vi "Initialize From Config.vi"(0 "Engine Data":T1={"Loop Info"={"Processor"=-2, "Priority"=0}, "Main Tag Data"={"Double"=[], "Single"=[], "I64"=[], "I32"=[], "I16"=[], "I8"=[], "U64"=[], "U32"=[], "U16"=[], "U8"=[], "Boolean"=[], "String"=[], "Array of Double"=[], "Array of Single"=[], "Array of I64"=[], "Array of I32"=[], "Array of I16"=[], "Array of I8"=[], "Array of U64"=[], "Array of U32"=[], "Array of U16"=[], "Array of U8"=[], "Array of Boolean"=[], "Array of String"=[]}, "Module Info"={"Tag Bus Modules"=[], "Execute?"=[], "Input Method Indices"=[], "Process Method Indices"=[], "Output Method Indices"=[], "Input Transfer Specifications"=[], "Parameter Transfer Specifications"=[], "Result Transfer Specifications"=[], "Output Transfer Specifications"=[], "Module Errors"=[], "Module Decimation"=[], "Module Decimation Indices"=[], "Error Queue"=refnum, "Module Error Configuration"=[], "Module Errors (n-1)"=[]}, "engine timing source"=refnum, "timing policy"=enum."nonblocking", "async execution info"={"Tag Bus Modules"=[], "Execute?"=[], "Input Method Indices"=[], "Process Method Indices"=[], "Output Method Indices"=[], "Input Transfer Specifications"=[], "Parameter Transfer Specifications"=[], "Result Transfer Specifications"=[], "Output Transfer Specifications"=[], "Module Errors"=[], "Module Decimation"=[], "Module Decimation Indices"=[], "Error Queue"=refnum, "Module Error Configuration"=[], "comm errors"=[], "Module Errors (n-1)"=[]}, "status reporting"={"late index (bool)"=-1, "late count (U32)"=-1, "current dt ns(U64)"=-1, "synchronous modules"=[], "asynchronous modules"=[]}}, 5 "Engine Configuration":refnum<class "Standard Engine Configuration.lvclass">, 7 "Modules":refnum<class "TBM module execution interface.lvclass">[](array[class]), 9 "Module Configurations":refnum<class "TBM module configuration.lvclass">[](array[class]), 11 "error in":errorcluster) -> (4 "Engine Data Out":T1={"Loop Info"={"Processor"=-2, "Priority"=0}, "Main Tag Data"={"Double"=[], "Single"=[], "I64"=[], "I32"=[], "I16"=[], "I8"=[], "U64"=[], "U32"=[], "U16"=[], "U8"=[], "Boolean"=[], "String"=[], "Array of Double"=[], "Array of Single"=[], "Array of I64"=[], "Array of I32"=[], "Array of I16"=[], "Array of I8"=[], "Array of U64"=[], "Array of U32"=[], "Array of U16"=[], "Array of U8"=[], "Array of Boolean"=[], "Array of String"=[]}, "Module Info"={"Tag Bus Modules"=[], "Execute?"=[], "Input Method Indices"=[], "Process Method Indices"=[], "Output Method Indices"=[], "Input Transfer Specifications"=[], "Parameter Transfer Specifications"=[], "Result Transfer Specifications"=[], "Output Transfer Specifications"=[], "Module Errors"=[], "Module Decimation"=[], "Module Decimation Indices"=[], "Error Queue"=refnum, "Module Error Configuration"=[], "Module Errors (n-1)"=[]}, "engine timing source"=refnum, "timing policy"=enum."nonblocking", "async execution info"={"Tag Bus Modules"=[], "Execute?"=[], "Input Method Indices"=[], "Process Method Indices"=[], "Output Method Indices"=[], "Input Transfer Specifications"=[], "Parameter Transfer Specifications"=[], "Result Transfer Specifications"=[], "Output Transfer Specifications"=[], "Module Errors"=[], "Module Decimation"=[], "Module Decimation Indices"=[], "Error Queue"=refnum, "Module Error Configuration"=[], "comm errors"=[], "Module Errors (n-1)"=[]}, "status reporting"={"late index (bool)"=-1, "late count (U32)"=-1, "current dt ns(U64)"=-1, "synchronous modules"=[], "asynchronous modules"=[]}}, 15 "error out":errorcluster)   [LabVIEW 2013, in "Standard Engine Runtime.lvclass"]
uses:
  Standard Engine Runtime.lvclass
  Engine Data.ctl
  <vilib>/NI/Module Timing Source/timing source/TBM timing source.lvclass
  Configuration/Loop Info.ctl
  <vilib>/NI/Tag Bus/table/data table.ctl
  Module Execution Info.ctl
  <vilib>/NI/Tag Bus Module Framework/runtime/TBM module execution interface.lvclass
  Data Table with Transfer Spec.ctl
  <vilib>/NI/Tag Bus/table/transfer specification.ctl
  <vilib>/NI/Tag Bus/tag/Data Type.ctl
  Configuration/Module Decimation.ctl
  Configuration/Module Error Configuration.ctl
  Configuration/Error Actions By Category.ctl
  <vilib>/NI/Tag Bus Module Framework/runtime/error classification.ctl
  Configuration/Error Actions.ctl
  Configuration/timing policy.ctl
  async execution info.ctl
  asynchronous process data.ctl
  async command notification.ctl
  <vilib>/NI/Tag Bus Module Framework/runtime/execution settings.ctl
  async error info.ctl
  status reporting data.ctl
  module status reporting.ctl
  Configuration/Standard Engine Configuration.lvclass
  <vilib>/NI/Tag Bus Module Framework/module configuration/TBM module configuration.lvclass
  Configuration/Standard Engine Configuration.lvclass/Standard Engine Configuration.ctl
  <vilib>/NI/Tag Bus Module Framework/root configuration/TBM configuration.lvclass/TBM configuration.ctl
  <vilib>/NI/Module Timing Source/standard timing source/ms timing source.lvclass
  <vilib>/NI/Module Timing Source/usec timing source/usec timing source.lvclass
  <vilib>/NI/Module Timing Source/scan engine timing source/scan engine timing source.lvclass
  <vilib>/NI/Module Timing Source/timing source/TBM timing source.lvclass/TBM timing source.ctl
  <vilib>/NI/Module Execution Interface/Engine Configuration/engine configuration.lvclass/engine configuration.ctl
  <vilib>/NI/Tag Bus/dictionary/data dictionary.lvclass/data dictionary.ctl
  <vilib>/NI/Tag Bus/dictionary/lookup polymorphs/locate I32.vi
  Configuration/Read timing policy.vi
  Configuration/Read Timing Source Type.vi
  Configuration/Read Processor.vi
  Configuration/Read Master Timing Module.vi
  <vilib>/NI/Tag Bus/dictionary/search/find data index.vi
  <vilib>/NI/Tag Bus/dictionary/search/search string list.vi
  Configuration/Read Timing Source dt.vi
  <vilib>/NI/Tag Bus Module Framework/root configuration/create GUID.vi
  Configuration/Find Module Specific Config.vi
  <vilib>/Utility/error.llb/Error Cluster From Error Code.vi
  <vilib>/NI/Tag Bus/dictionary/tag not found.vi
  <vilib>/NI/Tag Bus/tag/tag descriptor.lvclass
  <vilib>/Utility/RT CPU pool selections.ctl
  <vilib>/NI/Tag Bus/dictionary/data dictionary.lvclass
  <vilib>/NI/Module Execution Interface/Engine Configuration/engine configuration.lvclass
  <vilib>/NI/Module Execution Interface/Engine Runtime/Engine Runtime Interface.lvclass
  <vilib>/NI/Tag Bus Module Framework/root configuration/TBM configuration.lvclass
  <vilib>/NI/Tag Bus/table/data table.lvlib
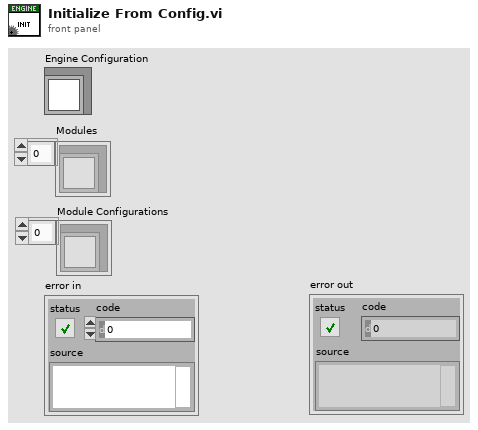
[diagram p1: front panel]
types:
  T1 = typedef "Standard Engine Runtime.lvclass/Engine Data.ctl" = cluster{"Loop Info":T2, "Main Tag Data":T3, "Module Info":T4, "engine timing source":refnum<class "TBM timing source.lvclass">, "timing policy":T13, "async execution info":T14, "status reporting":T17}
  T2 = typedef "Standard Engine Configuration.lvclass/Loop Info.ctl" = cluster{"Processor":i32, "Priority":i32}
  T3 = typedef "tag bus.lvlib/data table.lvlib/data table.ctl" = cluster{"Double":dbl[], "Single":sgl[], "I64":i64[], "I32":i32[], "I16":i16[], "I8":i8[], "U64":u64[], "U32":u32[], "U16":u16[], "U8":u8[], "Boolean":bool[], "String":string[], "Array of Double":cluster{"DBL Array":dbl[]}[], "Array of Single":cluster{"SGL Array":sgl[]}[], "Array of I64":cluster{"I64 Array":i64[]}[], "Array of I32":cluster{"I32 Array":i32[]}[], "Array of I16":cluster{"I16 Array":i16[]}[], "Array of I8":cluster{"I8 Array":i8[]}[], "Array of U64":cluster{"U64 Array":u64[]}[], "Array of U32":cluster{"U32 Array":u32[]}[], "Array of U16":cluster{"U16 Array":u16[]}[], "Array of U8":cluster{"U8 Array":u8[]}[], "Array of Boolean":cluster{"Boolean Array":bool[]}[], "Array of String":cluster{"String Array":string[]}[]}
  T4 = typedef "Standard Engine Runtime.lvclass/Module Execution Info.ctl" = cluster{"Tag Bus Modules":refnum<class "TBM module execution interface.lvclass">[], "Execute?":bool[], "Input Method Indices":i32[], "Process Method Indices":i32[], "Output Method Indices":i32[], "Input Transfer Specifications":T5[], "Parameter Transfer Specifications":T5[], "Result Transfer Specifications":T5[], "Output Transfer Specifications":T5[], "Module Errors":errorcluster[], "Module Decimation":T8[], "Module Decimation Indices":i32[], "Error Queue":refnum<queue>, "Module Error Configuration":T9[], "Module Errors (n-1)":errorcluster[]}
  T5 = typedef "Standard Engine Runtime.lvclass/Data Table with Transfer Spec.ctl" = cluster{"Data Table":T3, "Transfer Specification":T6[]}
  T6 = typedef "tag bus.lvlib/data table.lvlib/transfer specification.ctl" = cluster{"data type":T7, "sink indices":i32[], "source indices":i32[]}
  T7 = typedef "tag bus.lvlib/tag descriptor.lvclass/Data Type.ctl" = enum16{"Double", "Single", "I64", "I32", "I16", "I8", "U64", "U32", "U16", "U8", "Boolean", "String", "Array of Double", "Array of Single", "Array of I64", "Array of I32", "Array of I16", "Array of I8", "Array of U64", "Array of U32", "Array of U16", "Array of U8", "Array of Boolean", "Array of String"}
  T8 = typedef "Standard Engine Configuration.lvclass/Module Decimation.ctl" = cluster{"Decimation":u16, "Offset":u16}
  T9 = typedef "Standard Engine Configuration.lvclass/Module Error Configuration.ctl" = cluster{"Module Error Configuration":T10[]}
  T10 = typedef "Standard Engine Configuration.lvclass/Error Actions By Category.ctl" = cluster{"error classification":T11, "Error Actions":T12[]}
  T11 = typedef "TBM module execution interface.lvclass/error classification.ctl" = enum16{"unknown", "none", "trivial", "recoverable", "critical"}
  T12 = typedef "Standard Engine Configuration.lvclass/Error Actions.ctl" = enum16{"Clear", "Notify", "Stop Component", "Stop Engine", "Safe State", "Attempt Recovery"}
  T13 = typedef "Standard Engine Configuration.lvclass/timing policy.ctl" = enum16{"strict determinism", "nonblocking", "nondeterministic inline"}
  T14 = typedef "Standard Engine Runtime.lvclass/async execution info.ctl" = cluster{"Tag Bus Modules":T15[], "Execute?":bool[], "Input Method Indices":i32[], "Process Method Indices":i32[], "Output Method Indices":i32[], "Input Transfer Specifications":T5[], "Parameter Transfer Specifications":T5[], "Result Transfer Specifications":T5[], "Output Transfer Specifications":T5[], "Module Errors":errorcluster[], "Module Decimation":T8[], "Module Decimation Indices":i32[], "Error Queue":refnum<queue>, "Module Error Configuration":T9[], "comm errors":errorcluster[], "Module Errors (n-1)":errorcluster[]}
  T15 = typedef "Standard Engine Runtime.lvclass/asynchronous process data.ctl" = cluster{"thread reference":refnum<vi>, "cmd notification":refnum<k33>, "execution period (ms)":i32, "input from component":refnum<queue>, "input to component":refnum<queue>, "output from component":refnum<queue>, "output to component":refnum<queue>, "process input from component":refnum<queue>, "process input to component":refnum<queue>, "process result from component":refnum<queue>, "process result to component":refnum<queue>, "execution settings":T16, "error fifo":refnum<k33>}
  T16 = typedef "TBM module execution interface.lvclass/execution settings.ctl" = cluster{"reads inputs":bool, "processes data":bool, "writes outputs":bool}
  T17 = typedef "Standard Engine Runtime.lvclass/status reporting data.ctl" = cluster{"late index (bool)":i32, "late count (U32)":i32, "current dt ns(U64)":i32, "synchronous modules":T18[], "asynchronous modules":T18[]}
  T18 = typedef "Standard Engine Runtime.lvclass/module status reporting.ctl" = cluster{"module index":i32, "error tag (I32)":i32}
  T19 = typedef "Standard Engine Configuration.lvclass/Supported Timing Sources.ctl" = enum16{"Use Module Timing Source", "1 kHz Clock", "1 MHz Clock", "Synchronize to Scan Engine"}
  T20 = cluster{"execution order priority":i32, "module index":i32}
  T21 = typedef "engine configuration.lvclass/Module Mappings.ctl" = cluster{"Owning ID":string, "Input Mappings":T22[], "Process Parameter Mappings":T22[], "Process Results Mappings":T22[], "Output Mappings":T22[]}
  T22 = typedef "tag bus.lvlib/data table.lvlib/mapping specification.ctl" = cluster{"data type":T7, "mappings":T23[]}
  T23 = typedef "tag bus.lvlib/data table.lvlib/mapping.ctl" = cluster{"sink name":string, "source name":string}
  T24 = typedef "TBM channel.lvclass/data tables.ctl" = cluster{"input data":T25, "processing parameter":T25, "processing result":T25, "output data":T25}
  T25 = typedef "tag bus.lvlib/dictionary table pair.ctl" = cluster{"data dictionary":refnum<class "data dictionary.lvclass">, "data table":T3}
  T26 = typedef "Standard Engine Configuration.lvclass/timing reporting tags.ctl" = cluster{"late index (bool)":string, "late count index (U32)":string, "current dt ns(U64)":string}
  T27 = typedef "NI_Real-Time Target Support.lvlib/RT CPU pool selections.ctl" = enum16{"System & Timed Structures", "System", "Timed Structures", "Reserved"}
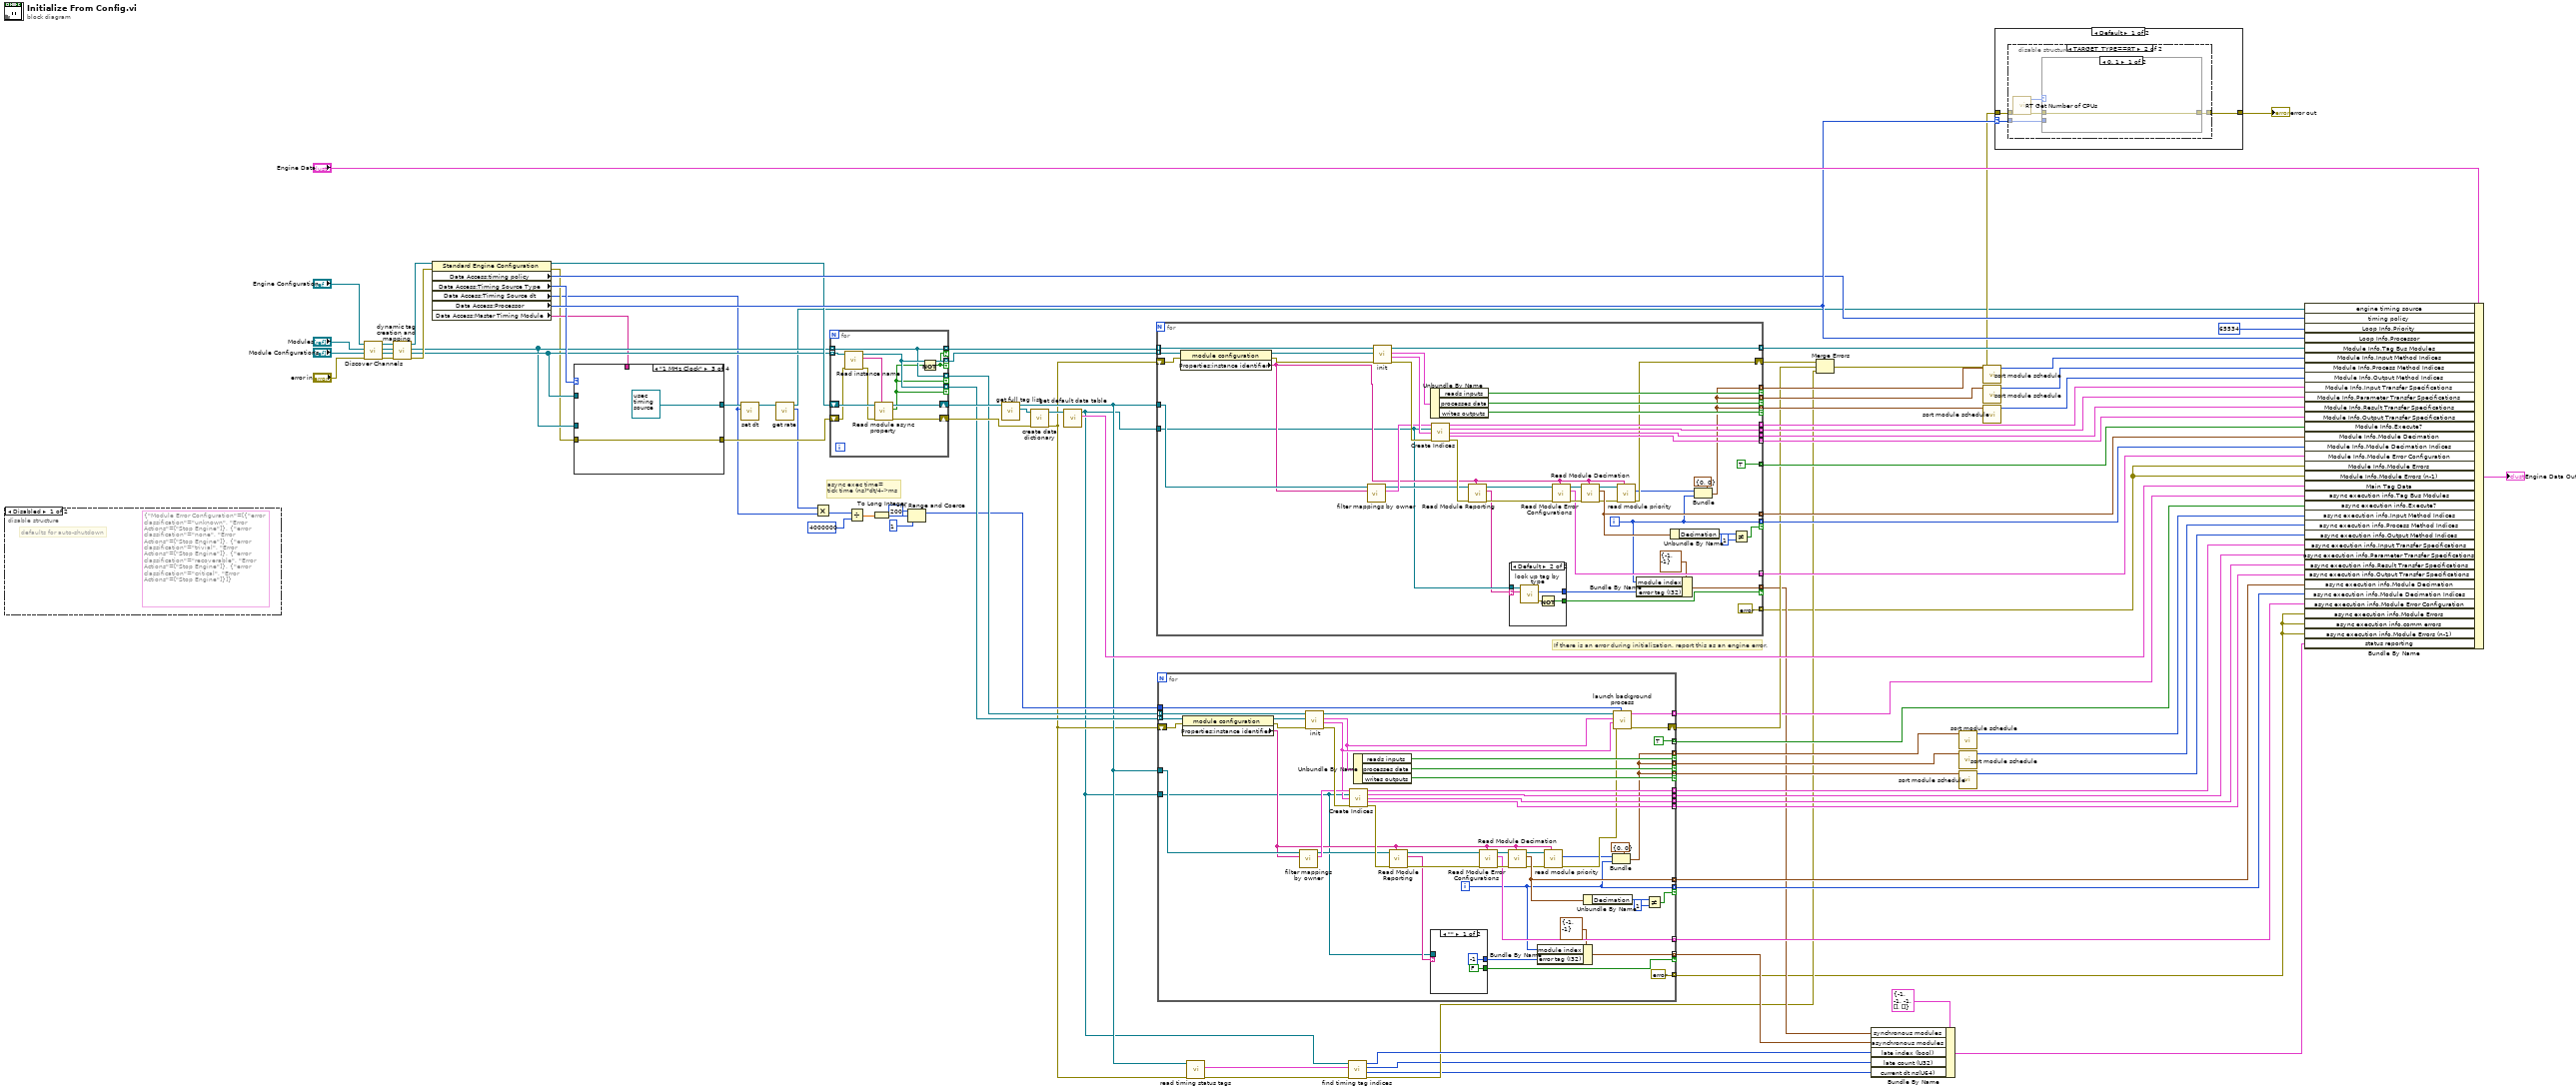
[diagram p0: block diagram]
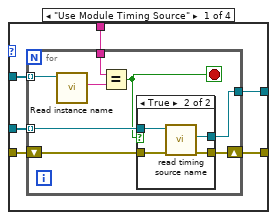
[diagram p2: hidden frame]
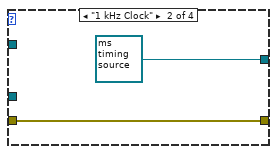
[diagram p4: hidden frame]
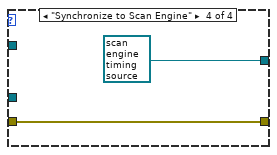
[diagram p5: hidden frame]
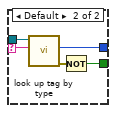
[diagram p6: hidden frame]
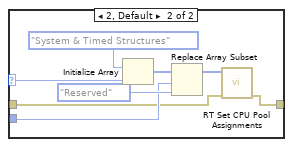
[diagram p9: hidden frame]
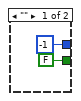
[diagram p11: hidden frame]
diagram:
  # "async exec time=\ntick time (ns)*dt/4->ms"
  # "If there is an error during initialization, report this as an engine error."
  n1 = disable-structure shown="Disabled" {
    frame Disabled {
      (unwired) T9 {"Module Error Configuration"=[{"error classification"=enum."unknown", "Error Actions"=[enum."Stop Engine"]}, {"error classification"=enum."none", "Error Actions"=[enum."Stop Engine"]}, {"error classification"=enum."trivial", "Error Actions"=[enum."Stop Engine"]}, {"error classification"=enum."recoverable", "Error Actions"=[enum."Stop Engine"]}, {"error classification"=enum."critical", "Error Actions"=[enum."Stop Engine"]}]} ("Module Error Configuration")
      # "defaults for auto-shutdown"
    }
    frame Enabled {
    }
  }
  n2 = call <vilib>:"Discover Channels.vi"("error in (no error)"="error in", "module configurations"="Module Configurations", "modules"="Modules", "engine configuration"="Engine Configuration") -> ("error out"=w76:errorcluster, "module configurations out"=w77:refnum<class "TBM module configuration.lvclass">[], "modules out"=w78:refnum<class "TBM module execution interface.lvclass">[], "engine configuration out"=w79:refnum<class "Standard Engine Configuration.lvclass">)  [unwired: 4 in]
  n3 = call <vilib>:"dynamic tag creation and mapping.vi"("error in"=w76, "module configurations"=w77, "modules"=w78, "engine configuration in"=w79) -> ("error out"=w70:errorcluster, "module configurations out"=w32:refnum<class "TBM module configuration.lvclass">[], "modules out"=w31:refnum<class "TBM module execution interface.lvclass">[], "engine configuration out"=w71:refnum<class "Standard Engine Configuration.lvclass">)  [unwired: 4 in]
  n4 = property class="Standard Engine Configuration"(reference=w71, error in=w70) -> (reference out=w57:refnum<class "Standard Engine Configuration.lvclass">, error out=w28:errorcluster, "Data Access:timing policy"=w58:T13, "Data Access:Timing Source Type"=w33:T19, "Data Access:Timing Source dt"=w23:u32, "Data Access:Processor"=w65:i32, "Data Access:Master Timing Module"=w30:string)
  n5 = case shown="\"1 MHz Clock\"" w33 {
    tunnel: [w95 refnum<class "ms timing source.lvclass"> refnum ("ms timing source.lvclass") refnum<class "usec timing source.lvclass"> refnum ("usec timing source.lvclass") refnum<class "scan engine timing source.lvclass"> refnum ("scan engine timing source.lvclass")] -> w27
    tunnel: w32 -> [w98 _ _ _]
    tunnel: w31 -> [w97 _ _ _]
    tunnel: w30 -> [w96 _ _ _]
    tunnel: [w94 w112 w114 w116] -> w29
    tunnel: w28 -> [w93 w112 w114 w116]
    frame "Use Module Timing Source" {
      n6 = for {
        tunnel: w98 -> [w106] mode=indexing
        tunnel: w97 -> [w103] mode=indexing
        tunnel: w96 -> [w104]
        tunnel: [w101] -> w95
        shift-right: [w100] -> w94
        shift-left: w93 -> [w99]
        stop <- w102 stop-if-true
        n7 = call <vilib>:"Read instance name.vi"("configuration in"=w106) -> ("instance id"=w105:string)  [unwired: 8 in, 2 out]
        n8 = Equal?(x=w104, y=w105) -> (x = y?=w102:bool)
        n9 = case shown="True" w102 {
          tunnel: w103 -> [_ w111]
          tunnel: [_ w110] -> w101
          tunnel: [w107 w109] -> w100
          tunnel: w99 -> [w107 w108]
          frame False {
          }
          frame True {
            n10 = call-dynamic "read timing source name.vi"("error in"=w108, "module in"=w111) -> ("error out"=w109:errorcluster, "timing source"=w110:refnum<class "TBM timing source.lvclass">)  [unwired: 7 in, 1 out]
          }
        }
      }
    }
    frame "1 kHz Clock" {
    }
    frame "1 MHz Clock" {
    }
    frame "Synchronize to Scan Engine" {
    }
  }
  n11 = call <vilib>:"set dt.vi"("dt"=w23, "timing source in"=w27) -> ("timing source out"=w26:refnum<class "TBM timing source.lvclass">)  [unwired: 9 in]
  n12 = call-dynamic "get rate.vi"("timing source in"=w26) -> ("period (ns)"=w24:i64, "timing source out"=w25:refnum<class "TBM timing source.lvclass">)  [unwired: 8 in, 1 out]
  n13 = Multiply(x=w24, y=w23) -> (x*y=w22:i64)
  n14 = for {
    tunnel: w32 -> [w128] mode=indexing
    tunnel: w31 -> [w123] mode=indexing
    shift-right: [w125] -> w56
    shift-left: w57 -> [w126]
    tunnel: [w124] -> w54 mode=indexing if=w119
    tunnel: [w123] -> w55 mode=indexing if=w119
    tunnel: [w124] -> w51 mode=indexing if=w118
    tunnel: [w123] -> w52 mode=indexing if=w118
    shift-right: [w122] -> w53
    shift-left: w29 -> [w120]
    n15 = call <vilib>:"Read instance name.vi"("error in"=w120, "configuration in"=w128) -> ("error out"=w121:errorcluster, "instance id"=w127:string, "configuration out"=w124:refnum<class "TBM module configuration.lvclass">)  [unwired: 7 in]
    n16 = call "Read module async property.vi"("Module ID"=w127, "error in"=w121, "Standard Engine Repo Data in"=w126) -> ("error out"=w122:errorcluster, "async?"=w118:bool, "Standard Engine Repo Data out"=w125:refnum<class "Standard Engine Configuration.lvclass">)  [unwired: 6 in]
    n17 = Not(x=w118) -> (.not. x?=w119:bool)
  }
  n18 = Divide(x=w22, y=i64 4000000) -> (x/y=w20:dbl)
  n19 = To Long Integer(number=w20) -> (32bit integer=w19:i32)
  n20 = In Range and Coerce(upper limit=200, x=w19, lower limit=1) -> (coerced(x)=w18:i32)  [unwired: 1 out]
  n21 = call <vilib>:"get full tag list.vi"("engine configuration in"=w56) -> ("tag list"=w69:refnum<class "tag descriptor.lvclass">[], "engine configuration out"=w11:refnum<class "Standard Engine Configuration.lvclass">)  [unwired: 9 in]
  n22 = call <vilib>:"create data dictionary.vi"("error in"=w53, "system tags"=w69) -> ("error out"=w10:errorcluster, "data dictionary"=w68:refnum<class "data dictionary.lvclass">)  [unwired: 8 in]
  n23 = call <vilib>:"get default data table.vi"("data dictionary in"=w68) -> ("default data table"=w80:T3, "data dictionary out"=w7:refnum<class "data dictionary.lvclass">)  [unwired: 9 in]
  n24 = for {
    tunnel: w54 -> [w158] mode=indexing
    shift-right: [w147] -> w84
    shift-left: w10 -> [w154]
    tunnel: w55 -> [w173] mode=indexing
    tunnel: [w152] -> w92 mode=indexing
    tunnel: [w144] -> w59 mode=indexing if=w172
    tunnel: [w144] -> w62 mode=indexing if=w171
    tunnel: [w144] -> w64 mode=indexing if=w170
    tunnel: [w169] -> w90 mode=indexing
    tunnel: [w168] -> w89 mode=indexing
    tunnel: [w167] -> w88 mode=indexing
    tunnel: [w166] -> w87 mode=indexing
    tunnel: [TRUE] -> w86 mode=indexing
    tunnel: [w133] -> w85 mode=indexing if=w162
    tunnel: [w149] -> w81 mode=indexing
    tunnel: [w157] -> w82 mode=indexing
    tunnel: [errorcluster {"status"=FALSE, "code"=0, "source"=""} ("error constant")] -> w2 mode=indexing
    tunnel: w7 -> [w132]
    tunnel: w11 -> [w141]
    tunnel: [w134] -> w14 mode=indexing if=w130
    i -> [w133]
    n25 = property class="module configuration"(reference=w158, error in=w154) -> (reference out=w155:refnum<class "TBM module configuration.lvclass">, error out=w142:errorcluster, "Properties:instance identifier"=w136:string)
    n26 = call <vilib>:"filter mappings by owner.vi"("owner"=w136, "engine configuration in"=w141) -> ("module mapping"=w153:T21, "engine configuration out"=w139:refnum<class "Standard Engine Configuration.lvclass">)  [unwired: 8 in]
    n27 = call-dynamic "init.vi"("error in"=w142, "module configuration"=w155, "module in"=w173) -> ("error out"=w165:errorcluster, "data allocations"=w159:T24, "execution settings"=w160:T16, "module out"=w152:refnum<class "TBM module execution interface.lvclass">)  [unwired: 5 in]
    n28 = Unbundle By Name(w160) -> ("reads inputs"=w172:bool, "processes data"=w171:bool, "writes outputs"=w170:bool)
    n29 = call "Create Indices.vi"("Component Mappings"=w153, "main data dictionary"=w132, "data description"=w159, "error in"=w165) -> ("Input Transfer Specification"=w169:T5, "Parameter Transfer Specifcation"=w168:T5, "Result Transfer Specifcation"=w167:T5, "Output Transfer Specifcation"=w166:T5, "error out"=w140:errorcluster)  [unwired: 7 in]
    n30 = call "Read Module Reporting.vi"("Module ID"=w136, "error in"=w140, "Standard Engine Repo Data in"=w139) -> ("error out"=w138:errorcluster, "error tag"=w129:string, "Standard Engine Repo Data out"=w137:refnum<class "Standard Engine Configuration.lvclass">)  [unwired: 6 in]
    n31 = case shown="Default" w129 {
      selector: w129 -> [_ w176]
      tunnel: w132 -> [_ w180]
      tunnel: [-1 ("index") w179] -> w131
      tunnel: [FALSE w177] -> w130
      frame "" {
      }
      frame Default {
        n32 = call-poly <vilib>:"look up tag by type.vi"("name"=w176, "data dictionary in"=w180) -> ("error out"=w178:errorcluster, "index"=w179:i32)  [unwired: 7 in, 1 out]
        n33 = Not(x=w178) -> (.not. x?=w177:bool)
      }
    }
    n34 = call "Read Module Error Configurations.vi"("Module ID"=w136, "error in"=w138, "Standard Engine Repo Data in"=w137) -> ("error out"=w150:errorcluster, "Module Error Configuration"=w149:T9, "Standard Engine Repo Data out"=w151:refnum<class "Standard Engine Configuration.lvclass">)  [unwired: 6 in]
    n35 = call "Read Module Decimation.vi"("Module ID"=w136, "error in"=w150, "Standard Engine Repo Data in"=w151) -> ("error out"=w148:errorcluster, "Module Decimation"=w157:T8, "Standard Engine Repo Data out"=w146:refnum<class "Standard Engine Configuration.lvclass">)  [unwired: 6 in]
    n36 = call "read module priority.vi"("Module ID"=w136, "error in"=w148, "Standard Engine Repo Data in"=w146) -> ("error out"=w147:errorcluster, "execution order priority"=w145:i32)  [unwired: 6 in, 1 out]
    n37 = Bundle By Name(cluster=T18 {"module index"=-1, "error tag (I32)"=-1} ("module status report"), "module index"=w133, "error tag (I32)"=w131) -> (w134:T18)
    n38 = Unbundle By Name(w157) -> ("Decimation"=w156:u16)
    n39 = Bundle(cluster=T20 {"execution order priority"=0, "module index"=0} ("priority cluster"), "execution order priority"=w145, "module index"=w133) -> (w144:T20)
    n40 = Not Equal?(x=w156, y=u16 1) -> (x != y?=w162:bool)
  }
  n41 = for {
    tunnel: w51 -> [w215] mode=indexing
    shift-right: [w197] -> w48
    shift-left: w10 -> [w211]
    tunnel: w52 -> [w228] mode=indexing
    tunnel: [w201] -> w45 mode=indexing if=w227
    tunnel: [w201] -> w46 mode=indexing if=w226
    tunnel: [w201] -> w47 mode=indexing if=w225
    tunnel: [w224] -> w40 mode=indexing
    tunnel: [w223] -> w39 mode=indexing
    tunnel: [w222] -> w38 mode=indexing
    tunnel: [w221] -> w37 mode=indexing
    tunnel: [TRUE] -> w43 mode=indexing
    tunnel: [w181] -> w35 mode=indexing if=w217
    tunnel: [w206] -> w50 mode=indexing
    tunnel: [w214] -> w36 mode=indexing
    tunnel: [errorcluster {"status"=FALSE, "code"=0, "source"=""} ("error constant")] -> w1 mode=indexing
    tunnel: w7 -> [w182]
    tunnel: w11 -> [w199]
    tunnel: [w196] -> w34 mode=indexing
    tunnel: w18 -> [w193]
    tunnel: [w186] -> w13 mode=indexing if=w184
    i -> [w181]
    n42 = property class="module configuration"(reference=w215, error in=w211) -> (reference out=w212:refnum<class "TBM module configuration.lvclass">, error out=w198:errorcluster, "Properties:instance identifier"=w188:string)
    n43 = call <vilib>:"filter mappings by owner.vi"("owner"=w188, "engine configuration in"=w199) -> ("module mapping"=w210:T21, "engine configuration out"=w190:refnum<class "Standard Engine Configuration.lvclass">)  [unwired: 8 in]
    n44 = call-dynamic "init.vi"("error in"=w198, "module configuration"=w212, "module in"=w228) -> ("error out"=w220:errorcluster, "data allocations"=w195:T24, "execution settings"=w194:T16, "module out"=w209:refnum<class "TBM module execution interface.lvclass">)  [unwired: 5 in]
    n45 = call "Create Indices.vi"("Component Mappings"=w210, "main data dictionary"=w182, "data description"=w195, "error in"=w220) -> ("Input Transfer Specification"=w224:T5, "Parameter Transfer Specifcation"=w223:T5, "Result Transfer Specifcation"=w222:T5, "Output Transfer Specifcation"=w221:T5, "error out"=w192:errorcluster)  [unwired: 7 in]
    n46 = Unbundle By Name(w194) -> ("reads inputs"=w227:bool, "processes data"=w226:bool, "writes outputs"=w225:bool)
    n47 = call "Read Module Reporting.vi"("Module ID"=w188, "error in"=w192, "Standard Engine Repo Data in"=w190) -> ("error out"=w191:errorcluster, "error tag"=w183:string, "Standard Engine Repo Data out"=w189:refnum<class "Standard Engine Configuration.lvclass">)  [unwired: 6 in]
    n48 = case shown="\"\"" w183 {
      selector: w183 -> [_ w231]
      tunnel: w182 -> [_ w235]
      tunnel: [-1 ("index") w234] -> w185
      tunnel: [FALSE w232] -> w184
      frame "" {
      }
      frame Default {
        n49 = call-poly <vilib>:"look up tag by type.vi"("name"=w231, "data dictionary in"=w235) -> ("error out"=w233:errorcluster, "index"=w234:i32)  [unwired: 7 in, 1 out]
        n50 = Not(x=w233) -> (.not. x?=w232:bool)
      }
    }
    n51 = call "Read Module Error Configurations.vi"("Module ID"=w188, "error in"=w191, "Standard Engine Repo Data in"=w189) -> ("error out"=w207:errorcluster, "Module Error Configuration"=w206:T9, "Standard Engine Repo Data out"=w208:refnum<class "Standard Engine Configuration.lvclass">)  [unwired: 6 in]
    n52 = call "Read Module Decimation.vi"("Module ID"=w188, "error in"=w207, "Standard Engine Repo Data in"=w208) -> ("error out"=w205:errorcluster, "Module Decimation"=w214:T8, "Standard Engine Repo Data out"=w203:refnum<class "Standard Engine Configuration.lvclass">)  [unwired: 6 in]
    n53 = Bundle By Name(cluster=T18 {"module index"=-1, "error tag (I32)"=-1} ("module status report"), "module index"=w181, "error tag (I32)"=w185) -> (w186:T18)
    n54 = call "read module priority.vi"("Module ID"=w188, "error in"=w205, "Standard Engine Repo Data in"=w203) -> ("error out"=w204:errorcluster, "execution order priority"=w202:i32)  [unwired: 6 in, 1 out]
    n55 = Unbundle By Name(w214) -> ("Decimation"=w213:u16)
    n56 = Bundle(cluster=T20 {"execution order priority"=0, "module index"=0} ("priority cluster"), "execution order priority"=w202, "module index"=w181) -> (w201:T20)
    n57 = call "launch background process.vi"("execution period (ms)"=w193, "error in"=w204, "data allocations"=w195, "execution settings"=w194, "module runtime"=w209) -> ("error out"=w197:errorcluster, "async data"=w196:T15)  [unwired: 5 in]
    n58 = Not Equal?(x=w213, y=u16 1) -> (x != y?=w217:bool)
  }
  n59 = call "read timing status tags.vi"("error in"=w10, "Standard Engine Configuration in"=w11) -> ("error out"=w8:errorcluster, "timing reporting"=w9:T26)  [unwired: 7 in, 1 out]
  n60 = call "find timing tag indices.vi"("error in"=w8, "timing reporting"=w9, "data dictionary in"=w7) -> ("error out"=w5:errorcluster, "dt ns"=w4:i32, "late count"=w3:i32, "late boolean"=w6:i32)  [unwired: 5 in]
  n61 = Merge Errors(w84, w48, w5) -> (w49:errorcluster)
  n62 = Bundle By Name(cluster=T17 {"late index (bool)"=-1, "late count (U32)"=-1, "current dt ns(U64)"=-1, "synchronous modules"=[], "asynchronous modules"=[]} ("status reporting"), "synchronous modules"=w14, "asynchronous modules"=w13, "late index (bool)"=w6, "late count (U32)"=w3, "current dt ns(U64)"=w4) -> (w12:T17)
  n63 = call "sort module schedule.vi"("priority array"=w45) -> ("sorted module indices"=w44:i32[])  [unwired: 10 in]
  n64 = call "sort module schedule.vi"("priority array"=w46) -> ("sorted module indices"=w41:i32[])  [unwired: 10 in]
  n65 = call "sort module schedule.vi"("priority array"=w47) -> ("sorted module indices"=w42:i32[])  [unwired: 10 in]
  n66 = call "sort module schedule.vi"("priority array"=w59) -> ("sorted module indices"=w60:i32[])  [unwired: 10 in]
  n67 = call "sort module schedule.vi"("priority array"=w62) -> ("sorted module indices"=w61:i32[])  [unwired: 10 in]
  n68 = call "sort module schedule.vi"("priority array"=w64) -> ("sorted module indices"=w63:i32[])  [unwired: 10 in]
  n69 = case shown="Default" w65 {
    selector: w65 -> [w236 _]
    tunnel: w49 -> [w238 w254]
    tunnel: [w237 w254] -> w83
    frame Default {
      n70 = disable-structure shown="TARGET_TYPE==RT" {
        disable-tunnel: w238 -> [w239 w243]
        disable-tunnel: w236 -> [_ w241]
        disable-tunnel: [w239 w240] -> w237
        frame condition #0 (active) {
        }
        frame condition #1 {
          n71 = call <vilib>:"RT Get Number of CPUs.vi"("error in (no error)"=w243) -> ("error out"=w242:errorcluster, "# of CPUs"=w244:u32)  [unwired: 9 in]
          n72 = case shown="0, 1" w244 {
            selector: w244 -> [_ w252]
            tunnel: w242 -> [w245 w247]
            tunnel: w241 -> [_ w249]
            tunnel: [w245 w246] -> w240
            frame 0, 1 {
            }
            frame 2, Default {
              n73 = Initialize Array(RT_CPU_pool_selections."System & Timed Structures" ("Enum"), w252) -> (w251:T27[])
              n74 = Replace Array Subset(array=w251, new element=RT_CPU_pool_selections."Reserved" ("new element/subarray"), index=w249) -> (w248:T27[])
              n75 = call <vilib>:"RT Set CPU Pool Assignments.vi"("error in (no error)"=w247, "CPU pools"=w248) -> ("error out"=w246:errorcluster)  [unwired: 6 in, 3 out]
            }
          }
        }
      }
    }
    frame -2 {
    }
  }
  "error out" <- w83
  n76 = Bundle By Name(cluster="Engine Data", "engine timing source"=w25, "timing policy"=w58, "Loop Info.Priority"=65534, "Loop Info.Processor"=w65, "Module Info.Tag Bus Modules"=w92, "Module Info.Input Method Indices"=w60, "Module Info.Process Method Indices"=w61, "Module Info.Output Method Indices"=w63, "Module Info.Input Transfer Specifications"=w90, "Module Info.Parameter Transfer Specifications"=w89, "Module Info.Result Transfer Specifications"=w88, "Module Info.Output Transfer Specifications"=w87, "Module Info.Execute?"=w86, "Module Info.Module Decimation"=w82, "Module Info.Module Decimation Indices"=w85, "Module Info.Module Error Configuration"=w81, "Module Info.Module Errors"=w2, "Module Info.Module Errors (n-1)"=w2, "Main Tag Data"=w80, "async execution info.Tag Bus Modules"=w34, "async execution info.Execute?"=w43, "async execution info.Input Method Indices"=w44, "async execution info.Process Method Indices"=w41, "async execution info.Output Method Indices"=w42, "async execution info.Input Transfer Specifications"=w40, "async execution info.Parameter Transfer Specifications"=w39, "async execution info.Result Transfer Specifications"=w38, "async execution info.Output Transfer Specifications"=w37, "async execution info.Module Decimation"=w36, "async execution info.Module Decimation Indices"=w35, "async execution info.Module Error Configuration"=w50, "async execution info.Module Errors"=w1, "async execution info.comm errors"=w1, "async execution info.Module Errors (n-1)"=w1, "status reporting"=w12) -> (→"Engine Data Out":T1)
